vi "Configure Balance Unbalance Conversion.vi"(0 "VISA resource name":refnum<visa-resource-name>, 1 "Channel (1)":i32=1, 2 "Trace (1)":i32=1, 5 "Conversion State (F: Disable)":bool, 7 "Parameter (0:SSS)":u16(ring) items=["SSS", "SDS", "SSD", "SCS", "SSC", "SDD", "SCD", "SDC", "SCC", "Imbalance 1", "Imbalance 2", "Imbalance 3", "Imbalance 4", "CMRR1", "CMRR2"], 9 "Balance Device Type (0: Unbalance - Balance)":u16(ring) items=["Unbalance - Balance", "Balance - Balance", "Unbalance - Unbalance - Balance"], 11 "error in (no error)":errorcluster, 12 "Port 1 (1)":i32=1, 13 "Port 2 (1)":i32=1) -> (4 "VISA resource name out":refnum<visa-resource-name>, 15 "error out":errorcluster)   [LabVIEW 2011, in "Agilent ENA Series.lvlib"]
doc: "This VI configures balance unbalance conversion."
uses:
  Agilent ENA Series.lvlib
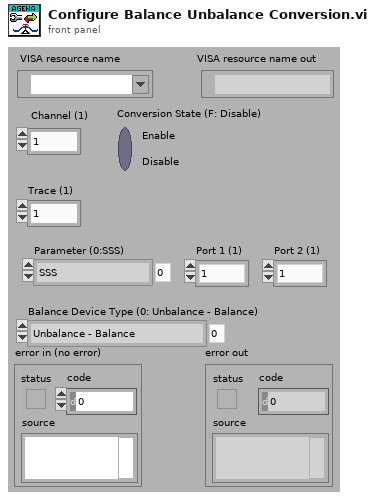
[diagram p1: front panel]
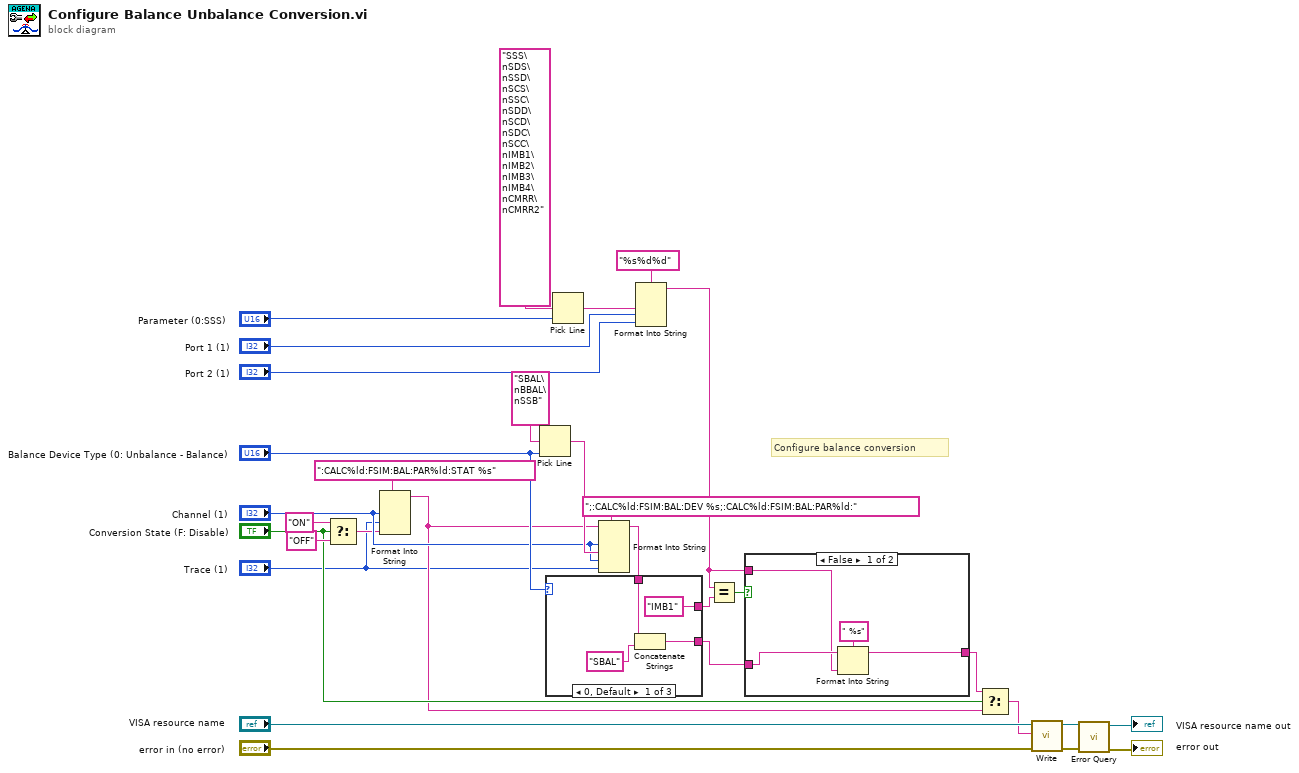
[diagram p0: block diagram]
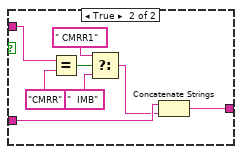
[diagram p2: hidden frame]
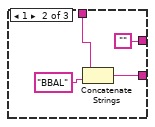
[diagram p3: hidden frame]
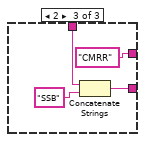
[diagram p4: hidden frame]
diagram:
  # "Configure balance conversion"
  n1 = Select(t="ON", s="Conversion State (F: Disable)", f="OFF") -> (s? t:f=w17:string)
  n2 = Format Into String(format string=":CALC%ld:FSIM:BAL:PAR%ld:STAT %s", "Channel (1)", "Trace (1)", w17) -> (resulting string=w18:string)  [unwired: 2 in, 1 out]
  n3 = Pick Line(multi-line string="SBAL\nBBAL\nSSB", line index="Balance Device Type (0: Unbalance - Balance)") -> (output string=w23:string)  [unwired: 1 in]
  n4 = Pick Line(multi-line string="SSS\nSDS\nSSD\nSCS\nSSC\nSDD\nSCD\nSDC\nSCC\nIMB1\nIMB2\nIMB3\nIMB4\nCMRR\nCMRR2", line index="Parameter (0:SSS)") -> (output string=w6:string)  [unwired: 1 in]
  n5 = Format Into String(format string=";:CALC%ld:FSIM:BAL:DEV %s;:CALC%ld:FSIM:BAL:PAR%ld:", initial string=w18, "Channel (1)", w23, "Channel (1)", "Trace (1)") -> (resulting string=w21:string)  [unwired: 1 in, 1 out]
  n6 = case shown="0, Default" "Balance Device Type (0: Unbalance - Balance)" {
    tunnel: w21 -> [w35 w37 w42]
    tunnel: [w33 w39 w43] -> w13
    tunnel: ["IMB1" "" "CMRR"] -> w15
    frame 0, Default {
      n7 = Concatenate Strings(w35, "SBAL" ("format string")) -> (w33:string)
    }
    frame 1 {
      n8 = Concatenate Strings(w37, "BBAL" ("format string")) -> (w39:string)
    }
    frame 2 {
      n9 = Concatenate Strings(w42, "SSB" ("format string")) -> (w43:string)
    }
  }
  n10 = Format Into String(format string="%s%d%d", w6, "Port 1 (1)", "Port 2 (1)") -> (resulting string=w3:string)  [unwired: 2 in, 1 out]
  n11 = Equal?(x=w3, y=w15) -> (x = y?=w14:bool)
  n12 = case shown="False" w14 {
    tunnel: w3 -> [w45 w54]
    tunnel: w13 -> [w47 w50]
    tunnel: [w44 w48] -> w12
    frame False {
      n13 = Format Into String(format string=" %s", initial string=w47, w45) -> (resulting string=w44:string)  [unwired: 1 in, 1 out]
    }
    frame True {
      n14 = Equal?(x=w54, y="CMRR") -> (x = y?=w53:bool)
      n15 = Select(t=" CMRR1", s=w53, f="  IMB") -> (s? t:f=w49:string)
      n16 = Concatenate Strings(w50, w49) -> (w48:string)
    }
  }
  n17 = Select(t=w12, s="Conversion State (F: Disable)", f=w18) -> (s? t:f=w20:string)
  n18 = call "Write.vi"("error in (no error)"="error in (no error)", "String ()"=w20, "VISA resource name"="VISA resource name") -> ("error out"=w10:errorcluster, "VISA resource name out"=w11:refnum<visa-resource-name>)  [unwired: 6 in, 1 out]
  n19 = call "Error Query.vi"("error in (no error)"=w10, "VISA resource name"=w11) -> ("error out"=→"error out":errorcluster, "VISA resource name out"=→"VISA resource name out":refnum<visa-resource-name>)  [unwired: 6 in, 2 out]
